vi "StateChangedEvent_GET.vi"(8 "error in":errorcluster, 11 "server in":refnum<class "RT FlexRIO Server TCP.lvclass">) -> (0 "error out":errorcluster, 2 "registered event":refnum<event-registration>, 3 "server out":refnum<class "RT FlexRIO Server TCP.lvclass">)   [LabVIEW 2017, in "RT FlexRIO Server TCP.lvclass"]
uses:
  RT FlexRIO Server TCP.lvclass
  Public/State.ctl
  RT FlexRIO Server TCP.lvclass/RT FlexRIO Server TCP.ctl
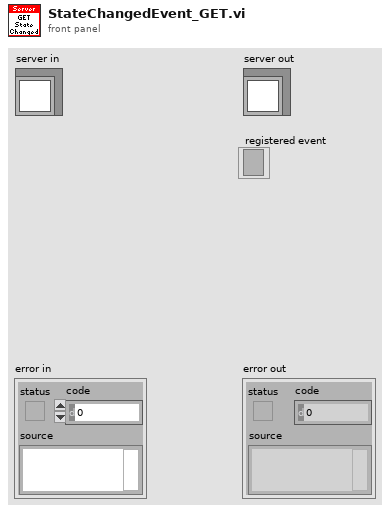
[diagram p1: front panel]
types:
  T1 = typedef "RT FlexRIO Server TCP.lvclass/SessionData.ctl" = cluster{"listener":refnum<k5>, "connection":refnum<k5>, "state":T2, "incoming":refnum<queue>, "outgoing":refnum<queue>, "state request":refnum<user-event>, "state changed":refnum<user-event>}
  T2 = typedef "RT FlexRIO Server TCP.lvclass/connection state.ctl" = enum16{"started", "connected", "stopped"}
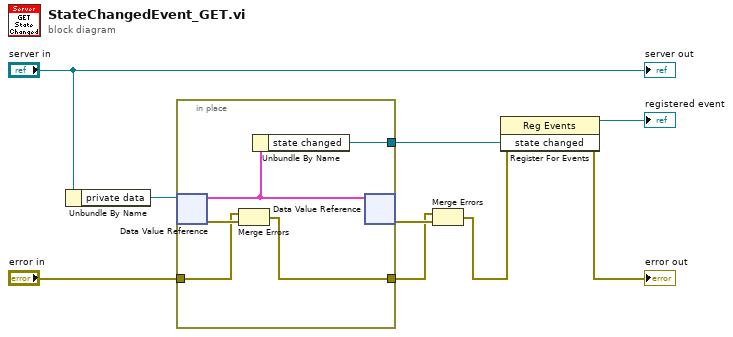
[diagram p0: block diagram]
diagram:
  n1 = Unbundle By Name("server in") -> ("private data"=w9:refnum<data-value>)
  n2 = in-place {
    in-place-border: "error in" -> [w10]
    in-place-border: [w14] -> w6
    in-place-border: [w12] -> w4
    n3 = in-place-dvr #1(w9) -> (w13:T1, w11:errorcluster)
    n4 = Merge Errors(w10, w11) -> (w14:errorcluster)
    n5 = Unbundle By Name(w13) -> ("state changed"=w12:refnum<user-event>)
    n6 = in-place-dvr #1(w13) -> (w7:errorcluster)  [unwired: 1 out]
  }
  n7 = Merge Errors(w6, w7) -> (w3:errorcluster)
  n8 = register-events(error in=w3, w4) -> (reference out=→"registered event":refnum<event-registration>, error out=→"error out":errorcluster)  [unwired: 1 in]
  "server out" <- "server in"
